vi "Charge_then_Discharge.vi"() -> ()   [LabVIEW 2020]
panel:
  out "PS error out":errorcluster
  out "PS Visa Out":refnum<visa-resource-name>
  in  "Discharge Current Cutoff":dbl
  in  "Discharge Current Setpoint (A)":dbl format="%#.6g"
  in  "Wait time":dbl
  in  "Batteryname":string
  in  "Charge Current Cutoff":dbl
  in  "Charge Current  Setpoint (A)":dbl format="%#.6g"
  in  "Battery Select":T1(ring)
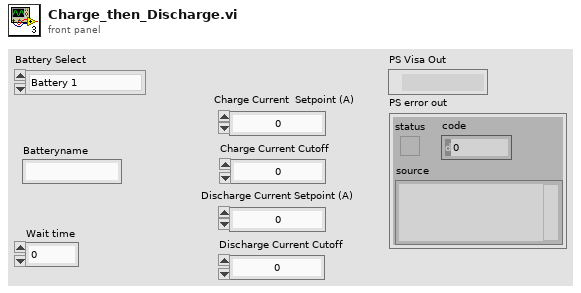
[diagram p1: front panel]
types:
  T1 = enum16{"Battery 1", "Battery 2", "Battery 3", "Battery 1&2", "Battery 1&3", "Battery 2&3", "Battery 1&2&3"}
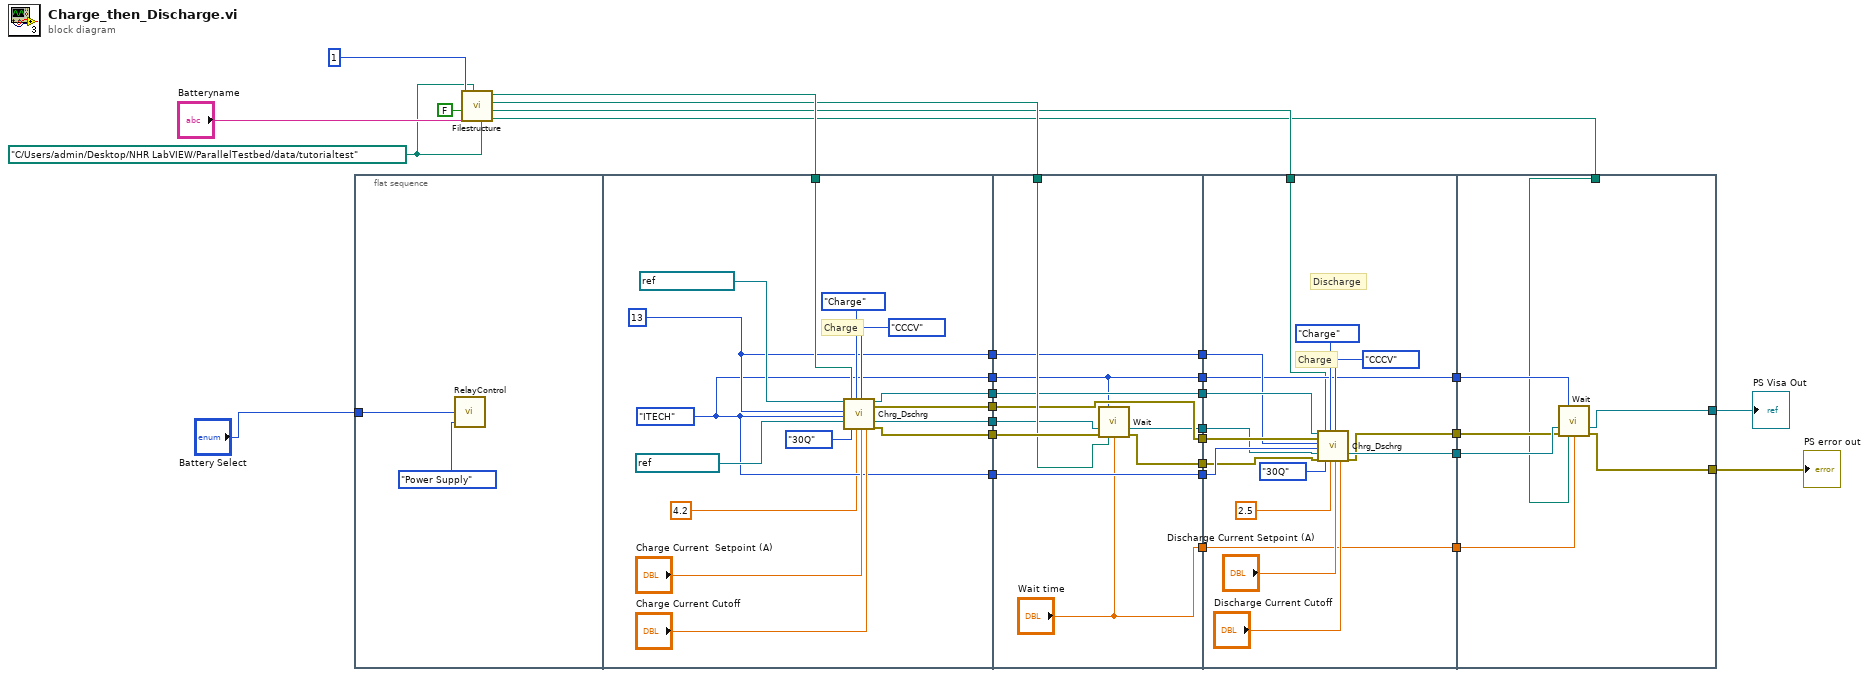
[diagram p0: block diagram]
diagram:
  w26 = path "C:/Users/admin/Desktop/NHR LabVIEW/ParallelTestbed/data/tutorialtest" ("Discharge filepath")
  n1 = flat-sequence {
    tunnel: "Battery Select" -> [w31]
    tunnel: w25 -> [w43]
    tunnel: [w40] -> w24
    tunnel: [w35] -> w23
    tunnel: [w37] -> w21
    tunnel: [w38] -> w19
    tunnel: [w36] -> w17
    tunnel: [w35] -> w15
    tunnel: [w34] -> w11
    tunnel: w24 -> [w58]
    tunnel: w23 -> [w49]
    tunnel: w22 -> [w57]
    tunnel: w21 -> [w56]
    tunnel: [w56] -> w20
    tunnel: w19 -> [w55]
    tunnel: [w55] -> w18
    tunnel: w17 -> [w54]
    tunnel: [w54] -> w16
    tunnel: w15 -> [w53]
    tunnel: [w53] -> w14
    tunnel: [w52] -> w13
    tunnel: [w51] -> w12
    tunnel: w11 -> [w50]
    tunnel: [w49] -> w8
    tunnel: ["Wait time"] -> w4
    tunnel: w20 -> [w72]
    tunnel: w18 -> [w71]
    tunnel: w16 -> [w70]
    tunnel: w14 -> [w69]
    tunnel: w13 -> [w68]
    tunnel: w12 -> [w67]
    tunnel: [w63] -> w10
    tunnel: [w62] -> w9
    tunnel: w8 -> [w61]
    tunnel: [w61] -> w7
    tunnel: w6 -> [w60]
    tunnel: w4 -> [w59]
    tunnel: [w59] -> w3
    tunnel: w10 -> [w82]
    tunnel: w9 -> [w81]
    tunnel: w7 -> [w80]
    tunnel: w5 -> [w79]
    tunnel: w3 -> [w78]
    tunnel: [w77] -> w2
    tunnel: [w76] -> w1
    frame #0 {
      n2 = call "RelayControl.vi"("NHR or Battery Analyzer"=enum16{"Battery Analyzer", "Power Supply"}."Power Supply", "Battery Select"=w31) -> ()  [unwired: 3 in]
    }
    frame #1 {
      w35 = enum16{"NHR", "ITECH"}."ITECH" ("PS type")
      w36 = 13 ("#DAQ outputs (1-13)")
      # "Charge"
      n3 = call "Chrg_Dschrg.vi"("Data Task in"=refnum<k21> "PTesbedTask", "#DAQ outputs (1-13)"=w36, "PS type"=w35, "PS VISA in"=refnum<visa-resource-name> "ITECH-PS3", "DischargeCyclePath"=w43, "Battery Type"=enum16{"30Q", "40T"}."30Q", "Charge/discharge"=enum8{"Charge", "Discharge"}."Charge", "Charge/Discharge Voltage Setpoint"=4.2, "CC or CCCV"=enum16{"CC", "CCCV"}."CCCV", "Current Setpoint"="Charge Current  Setpoint (A)", "Current Cutoff"="Charge Current Cutoff") -> ("data task out"=w37:refnum<k21>, "data task error out"=w38:errorcluster, "PS VIS resource name out"=w34:refnum<visa-resource-name>, "PS error out"=w40:errorcluster)  [unwired: 5 in]
    }
    frame #2 {
      n4 = call "Wait.vi"("PS type"=w49, "PS VISA in"=w50, "PS error in"=w58, "Wait Filepath"=w57, "Wait time"="Wait time") -> ("PS Visa Out"=w51:refnum<visa-resource-name>, "PS error out"=w52:errorcluster)  [unwired: 7 in, 2 out]
    }
    frame #3 {
      # "Charge"
      # "Discharge"
      n5 = call "Chrg_Dschrg.vi"("Data Task in"=w72, "data task error in"=w71, "#DAQ outputs (1-13)"=w70, "PS type"=w69, "PS VISA in"=w67, "PS error in"=w68, "DischargeCyclePath"=w60, "Battery Type"=enum16{"30Q", "40T"}."30Q", "Charge/discharge"=enum8{"Charge", "Discharge"}."Charge", "Charge/Discharge Voltage Setpoint"=2.5, "CC or CCCV"=enum16{"CC", "CCCV"}."CCCV", "Current Setpoint"="Discharge Current Setpoint (A)", "Current Cutoff"="Discharge Current Cutoff") -> ("PS VIS resource name out"=w63:refnum<visa-resource-name>, "PS error out"=w62:errorcluster)  [unwired: 3 in, 2 out]
    }
    frame #4 {
      n6 = call "Wait.vi"("PS type"=w80, "PS VISA in"=w82, "PS error in"=w81, "Wait Filepath"=w79, "Wait time"=w78) -> ("PS Visa Out"=w77:refnum<visa-resource-name>, "PS error out"=w76:errorcluster)  [unwired: 7 in, 2 out]
    }
  }
  n7 = call "Filestructure.vi"("Discharge filepath"=w26, "Batteryname"="Batteryname", "Charge filepath"=w26, "In for loop"=FALSE, "Starting Cycle"=1) -> ("DischargeWaitPath"=w5:path, "DischargeCyclePath"=w6:path, "ChargeWaitPath"=w22:path, "ChargeCyclePath"=w25:path)  [unwired: 2 in, 1 out]
  "PS Visa Out" <- w2
  "PS error out" <- w1
